vi "Radians to Degrees (Scalar DBL).vi"(3 "angle (rad)":dbl caption="角（弧度）") -> (1 "angle (deg)":dbl caption="角（角度）")   [LabVIEW 2011, in "NI_AngleManipulation.lvlib"]
doc: "Converts an angle from radians to degrees."
uses:
  <vilib>/Utility/AngleManip/NI_AngleManipulation.lvlib
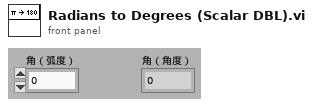
[diagram p1: front panel]
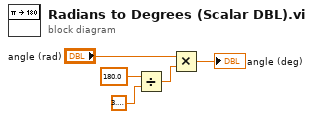
[diagram p0: block diagram]
diagram:
  n1 = Divide(x=180.0 ("y"), y=3.141592653589793) -> (x/y=w2:dbl)
  n2 = Multiply(x="angle (rad)", y=w2) -> (x*y=→"angle (deg)":dbl)
